vi "Simulated Thermocouple Main Page.vi"(8 "error in (no error)":errorcluster, 11 "Node Ptr":T2 format="%.0x") -> (0 "error out":errorcluster)   [LabVIEW 2011, in "Simulated Thermocouple Custom Device.lvlib"]
uses:
  Simulated Thermocouple Custom Device.lvlib
  <vilib>/NI Veristand/Custom Device API/Custom Device Item Ref.ctl
  TC Unit Selector.ctl
  Device Settings.ctl
  <vilib>/NI Veristand/Custom Device API/Get Item Property (Variant).vi
  <vilib>/NI Veristand/Custom Device API/Set Item Property (Variant).vi
  <vilib>/NI Veristand/Custom Device API/Custom Device API.lvlib
panel:
  in  "Physical Device":string
  in  "Temperature Units":T1 items=["Celcius", "Fahrenheit", "Kelvin", "Rankine"]
  in  "Output Update Rate [Hz]":dbl=25.0
  in  "Low Side Resistor\n(Ohms)":dbl=150.0 min=0.1 step=1.0
  in  "High Side Resistor\n(Ohms)":dbl=15000.0 min=0.1 step=1.0
  in  "Header 2":cluster{"Section Name":string}={"Section Name"="External Configuration"}
  in  "Header":cluster{"Section Name":string}={"Section Name"="Custom Device Item Settings"}
  in  "Description":string="This Custom Device will allow you to use your standard +/- 10 V Analog output hardware to simulate Thermocouples to your device under test.  Remaining channels can be configured as standard voltage or current outputs as allowed by the type of hardware being used.  \n\nThe basic concept is that a normal analog output channel can be brought to a lower scale using an external voltage divider.  The actual resistance values of the voltage divider used in your setup can be inputted below to ensure proper signal output.  Be sure the total resistance (R1+R2) is not too low, or the resulting current generated at a full scale 10V may exceed the ouput capability of the DAC used.  1KOhm or higher is a good rule of thumb.  R1 must also be approxmiately 10x R2 to get a deisired 100mV range useful to simulate thermocouples.  Ratios higher than this may clip the output signal below the full scale of the thermocouple being simulated.\n\nSimulated TC values will be updated at the fixed rate designated by Output Update Rate.  "
  in  "Name":string
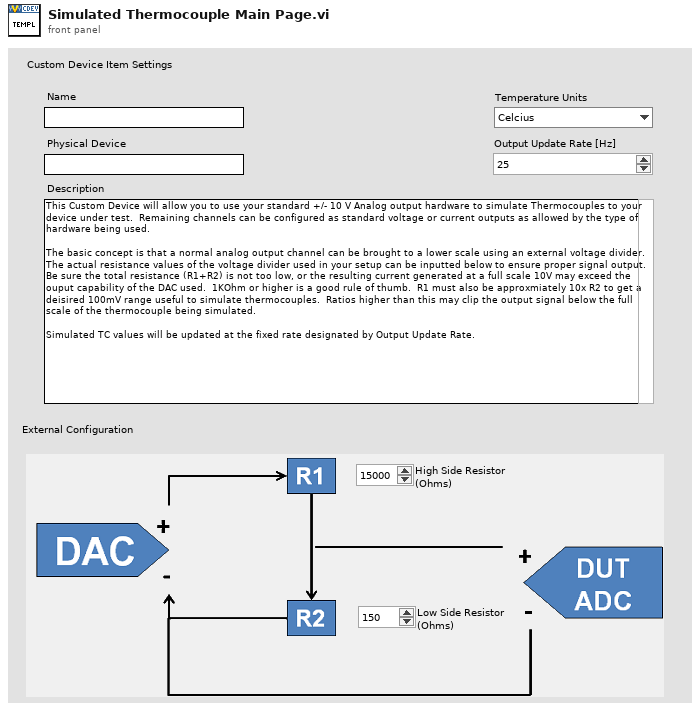
[diagram p1: front panel]
types:
  T1 = typedef "Simulated Thermocouple Custom Device.lvlib/TC Unit Selector.ctl" = u16
  T2 = typedef "Custom Device API.lvlib/Custom Device Item Ref.ctl" = u64
  T3 = typedef "Simulated Thermocouple Custom Device.lvlib/Device Settings.ctl" = cluster{"High Side Resistance (Ohms)":dbl, "Low Side Resistance (Ohms)":dbl, "Temperature Units":T1, "Update Rate":dbl, "Physical Device Name":string, "Device Channel Count":dbl}
  T4 = typedef "Custom Device API.lvlib/Custom Device Item Info.ctl" = cluster{"Name":string, "Is Channel":bool, "GUID":string}
  T5 = typedef "Custom Device API.lvlib/Custom Device Commands.ctl" = enum16{"Default", "Item renamed", "Shutdown", "Dynamic button pressed"}
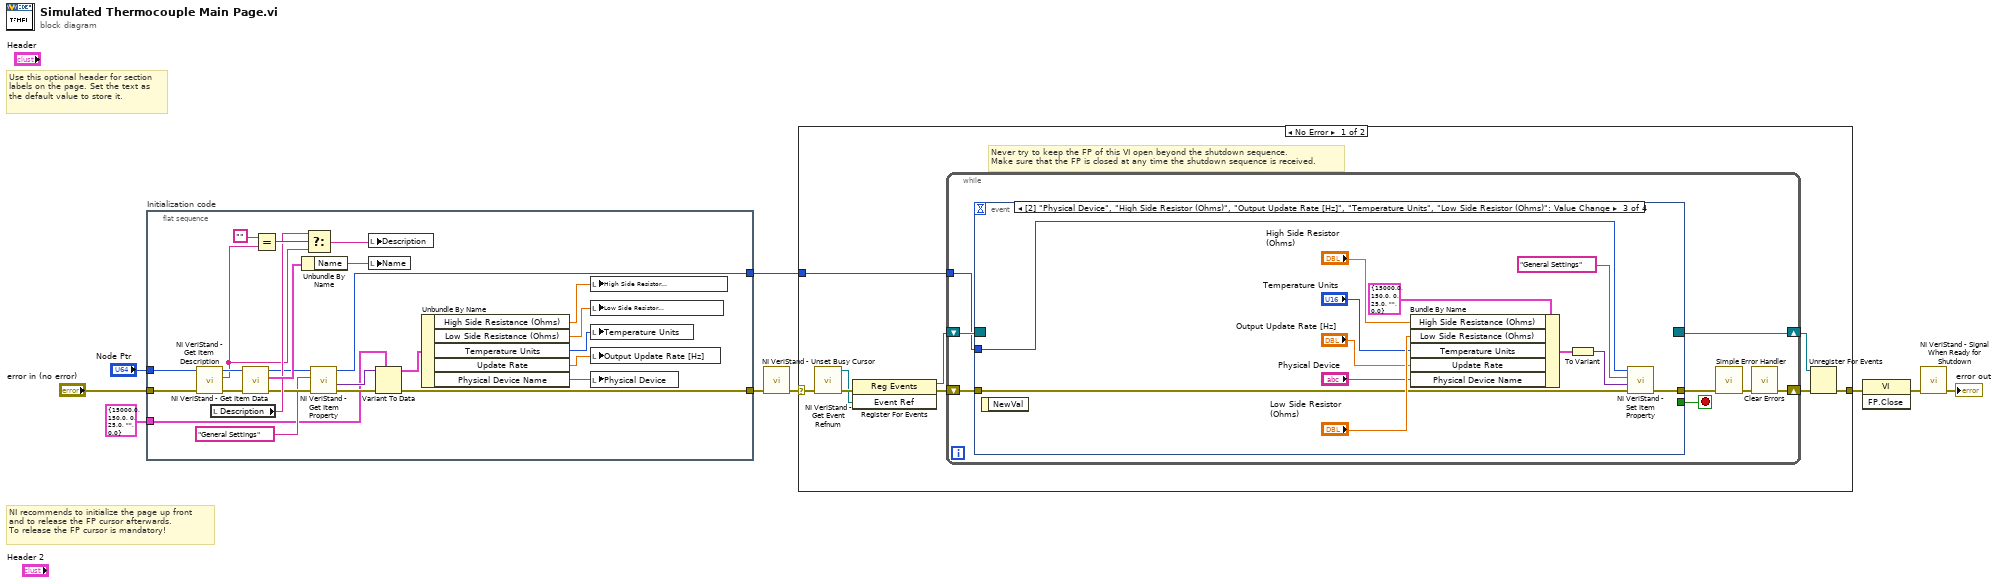
[diagram p0: block diagram]
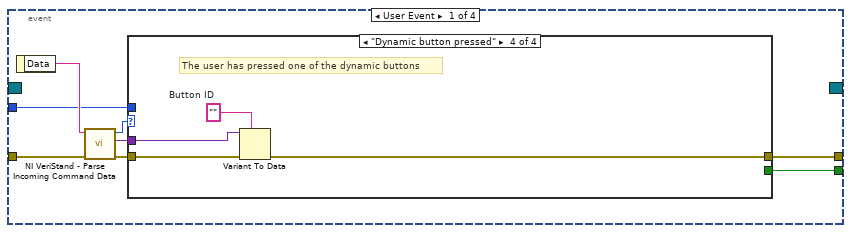
[diagram p2: hidden frame]
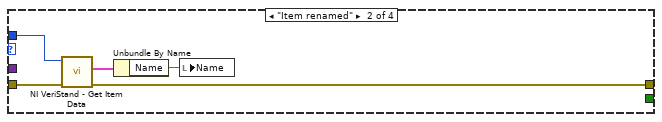
[diagram p4: hidden frame]
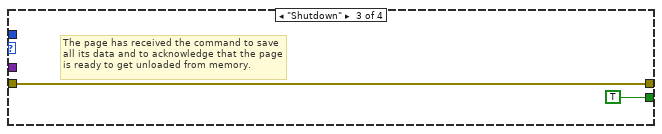
[diagram p5: hidden frame]
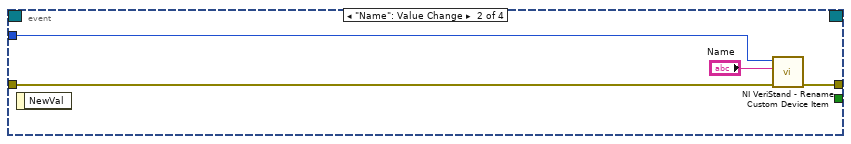
[diagram p6: hidden frame]
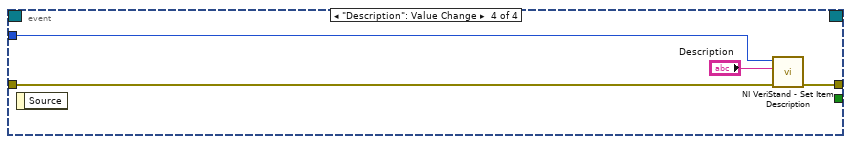
[diagram p7: hidden frame]
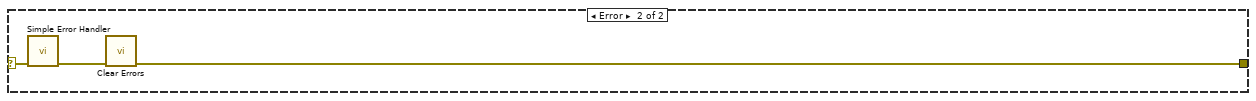
[diagram p8: hidden frame]
diagram:
  # "Use this optional header for section labels on the page. Set the text as the default value to store it."
  # "NI recommends to initialize the page up front\nand to release the FP cursor afterwards.\nTo release the FP cursor is mandatory!"
  n1 = flat-sequence "Initialization code" {
    tunnel: "error in (no error)" -> [w33]
    tunnel: "Node Ptr" -> [w32]
    tunnel: [w19] -> w5
    tunnel: [w10] -> w2
    tunnel: T3 {"High Side Resistance (Ohms)"=15000.0, "Low Side Resistance (Ohms)"=150.0, "Temperature Units"=0, "Update Rate"=25.0, "Physical Device Name"="", "Device Channel Count"=0.0} ("General Settings") -> [w17]
    frame #0 {
      n2 = call <vilib>:"NI VeriStand - Get Item Description.vi"("error in (no error)"=w33, "Item Ref in"=w32) -> ("error out"=w31:errorcluster, "Description"=w24:string, "Item Ref out"=w34:T2)  [unwired: 7 out]
      n3 = local read "Description"() -> (w26:string)
      n4 = call <vilib>:"NI VeriStand - Get Item Data.vi"("error in (no error)"=w31, "Item Ref in"=w34) -> ("error out"=w22:errorcluster, "Item Info"=w30:T4, "Item Ref out"=w23:T2)  [unwired: 7 out]
      n5 = Equal?(x="", y=w24) -> (x = y?=w28:bool)
      n6 = Unbundle By Name(w30) -> ("Name"=w29:string)
      n7 = Select(t=w26, s=w28, f=w24) -> (s? t:f=w25:string)
      n8 = call-poly <vilib>:"NI VeriStand - Get Item Property.vi"("error in (no error)"=w22, "Property Name"="General Settings", "Item Ref in"=w23) -> ("error out"=w20:errorcluster, "Value"=w18:variant, "Item Ref out"=w10:T2)  [unwired: 5 in, 1 out]
      n9 = local write "Description"(w25) -> ()
      n10 = local write "Name"(w29) -> ()
      n11 = Variant To Data(error in=w20, type=w17, Variant=w18) -> (data=w16:T3, error out=w19:errorcluster)
      n12 = Unbundle By Name(w16) -> ("High Side Resistance (Ohms)"=w15:dbl, "Low Side Resistance (Ohms)"=w14:dbl, "Temperature Units"=w13:T1, "Update Rate"=w12:dbl, "Physical Device Name"=w11:string)
      n13 = local write "High Side Resistor\n(Ohms)"(w15) -> ()
      n14 = local write "Low Side Resistor\n(Ohms)"(w14) -> ()
      n15 = local write "Temperature Units"(w13) -> ()
      n16 = local write "Output Update Rate [Hz]"(w12) -> ()
      n17 = local write "Physical Device"(w11) -> ()
    }
  }
  n18 = call <vilib>:"NI VeriStand - Unset Busy Cursor.vi"("error in (no error)"=w5) -> ("error out"=w4:errorcluster)  [unwired: 10 out]
  n19 = case shown="No Error" w4 {
    selector: w4 -> [w35 w94]
    tunnel: [w40 w92] -> w9
    tunnel: w2 -> [w36 _]
    frame No Error {
      # "Never try to keep the FP of this VI open beyond the shutdown sequence.\nMake sure that the FP is closed at any time the shutdown sequence is received."
      n20 = call <vilib>:"NI VeriStand - Get Event Refnum.vi"("error in (no error)"=w35) -> ("error out"=w43:errorcluster, "Event Ref"=w39:refnum<user-event>)  [unwired: 9 out]
      n21 = register-events(error in=w43, w39) -> (reference out=w37:refnum<event-registration>, error out=w38:errorcluster)  [unwired: 1 in]
      n22 = while {
        tunnel: w36 -> [w47]
        shift-right: [w44] -> w41
        shift-left: w38 -> [w50]
        shift-right: [w51] -> w42
        shift-left: w37 -> [w49]
        stop <- w48 stop-if-true
        n23 = event shown="[2] \"Physical Device\", \"High Side Resistor\n(Ohms)\", \"Output Update Rate [Hz]\", \"Temperature Units\", \"Low Side Resistor\n(Ohms)\": Value Change" {
          selector: w49 -> [_ _ _ _]
          dyn-events: [_ _ _ _] -> w51
          timeout: _ -> [_ _ _ _]
          tunnel: w50 -> [w59 w75 w80 w90]
          tunnel: [w55 _ _ _] -> w48
          tunnel: [w54 w74 w79 w89] -> w46
          tunnel: w47 -> [w53 w73 w82 w91]
          event User Event {
            n24 = event-data() -> ("Data"=w58:string)  [unwired: 1 out]
            n25 = call <vilib>:"NI VeriStand - Parse Incoming Command Data.vi"("error in (no error)"=w59, "Incoming data"=w58) -> ("error out"=w57:errorcluster, "Outgoing data"=w52:variant, "Action"=w56:T5)  [unwired: 7 out]
            n26 = case shown="\"Dynamic button pressed\"" w56 {
              tunnel: w57 -> [w60 w65 w66 w71]
              tunnel: [_ _ TRUE _] -> w55
              tunnel: [w60 w62 w66 w68] -> w54
              tunnel: w53 -> [_ w64 _ _]
              tunnel: w52 -> [_ _ _ w70]
              frame "Default", Default {
              }
              frame "Item renamed" {
                n27 = call <vilib>:"NI VeriStand - Get Item Data.vi"("error in (no error)"=w65, "Item Ref in"=w64) -> ("error out"=w62:errorcluster, "Item Info"=w63:T4)  [unwired: 8 out]
                n28 = Unbundle By Name(w63) -> ("Name"=w61:string)
                n29 = local write "Name"(w61) -> ()
              }
              frame "Shutdown" {
                # "The page has received the command to save all its data and to acknowledge that the page is ready to get unloaded from memory."
              }
              frame "Dynamic button pressed" {
                w69 = ""  # Button ID
                # "The user has pressed one of the dynamic buttons"
                n30 = Variant To Data(error in=w71, type=w69, Variant=w70) -> (error out=w68:errorcluster)  [unwired: 1 out]
              }
            }
          }
          event "Name": Value Change {
            n31 = event-data() -> ()  [unwired: 2 out]
            n32 = call <vilib>:"NI VeriStand - Rename Custom Device Item.vi"("error in (no error)"=w75, "New Name"="Name", "Item Ref in"=w73) -> ("error out"=w74:errorcluster)  [unwired: 8 out]
          }
          event "Physical Device", "High Side Resistor\n(Ohms)", "Output Update Rate [Hz]", "Low Side Resistor\n(Ohms)": Value Change {
            n33 = event-data() -> ()  [unwired: 2 out]
            n34 = Bundle By Name(cluster=T3 {"High Side Resistance (Ohms)"=15000.0, "Low Side Resistance (Ohms)"=150.0, "Temperature Units"=0, "Update Rate"=25.0, "Physical Device Name"="", "Device Channel Count"=0.0} ("General Settings"), "High Side Resistance (Ohms)"="High Side Resistor\n(Ohms)", "Low Side Resistance (Ohms)"="Low Side Resistor\n(Ohms)", "Temperature Units"="Temperature Units", "Update Rate"="Output Update Rate [Hz]", "Physical Device Name"="Physical Device") -> (w77:T3)
            n35 = To Variant(anything=w77) -> (Variant=w76:variant)
            n36 = call-poly <vilib>:"NI VeriStand - Set Item Property.vi"("error in (no error)"=w80, "Value"=w76, "Property Name"="General Settings", "Item Ref in"=w82) -> ("error out"=w79:errorcluster)  [unwired: 5 in, 2 out]
          }
          event "Description": Value Change {
            n37 = event-data() -> ()  [unwired: 2 out]
            n38 = call <vilib>:"NI VeriStand - Set Item Description.vi"("error in (no error)"=w90, "Description"="Description", "Item Ref in"=w91) -> ("error out"=w89:errorcluster)  [unwired: 8 out]
          }
        }
        n39 = call <vilib>:"Simple Error Handler.vi"("error in (no error)"=w46) -> ("error out"=w45:errorcluster)  [unwired: 1 in, 7 out]
        n40 = call <vilib>:"Clear Errors.vi"("error in (no error)"=w45) -> ("error out"=w44:errorcluster)  [unwired: 6 out]
      }
      n41 = Unregister For Events(event registration refnum=w42, error in=w41) -> (error out=w40:errorcluster)
    }
    frame Error {
      n42 = call <vilib>:"Simple Error Handler.vi"("error in (no error)"=w94) -> ("error out"=w93:errorcluster)  [unwired: 1 in, 7 out]
      n43 = call <vilib>:"Clear Errors.vi"("error in (no error)"=w93) -> ("error out"=w92:errorcluster)  [unwired: 6 out]
    }
  }
  n44 = invoke class="VI" method="FP.Close"(error in=w9) -> (error out=w8:errorcluster)  [unwired: 2 in, 2 out]
  n45 = call <vilib>:"NI VeriStand - Signal When Ready for Shutdown.vi"("error in (no error)"=w8) -> ("error out"=→"error out":errorcluster)  [unwired: 10 out]
